vi "TestFastLocalizeCPU.vi"() -> ()   [LabVIEW 2011]
uses:
  CpuTrackDLL.vi
panel:
  out "debug":T1(plugin-control)
  out "median":sgl
  out "xcorpos":cluster{"XCor X":sgl, "XCor Y":sgl}
  out "COM":cluster{"comX":sgl, "comY":sgl}
  out "Image":T1(plugin-control)
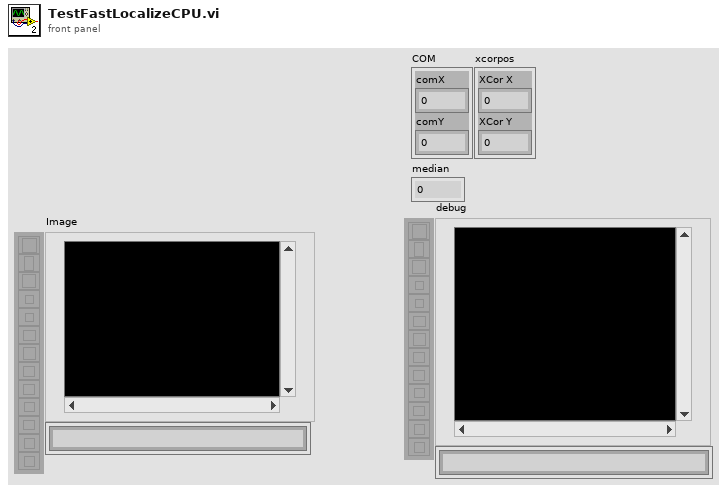
[diagram p1: front panel]
types:
  T1 = typedef "IMAQ Image.ctl" = refnum<image>
  T2 = typedef "Image Type" = u32
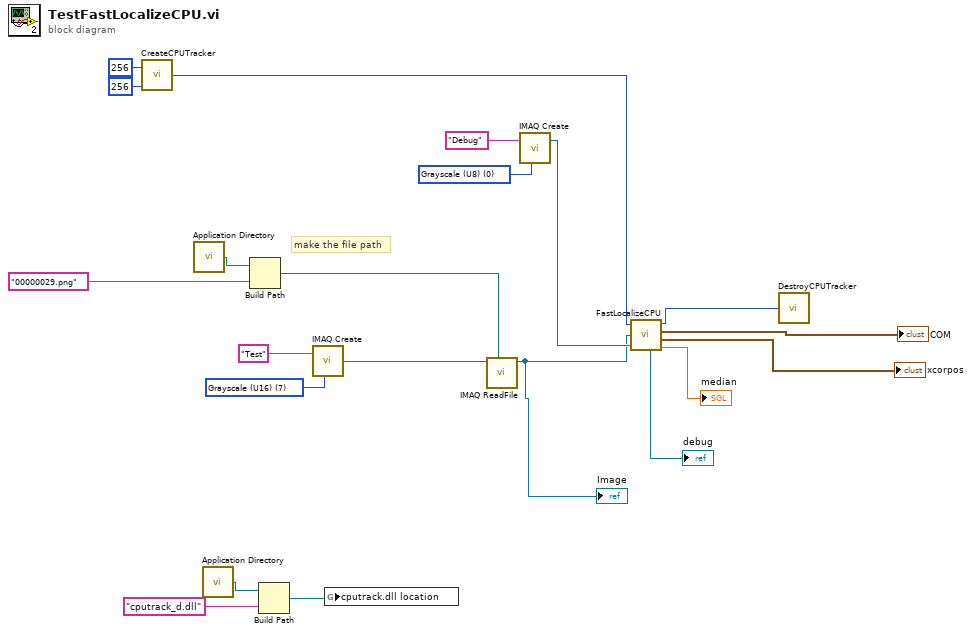
[diagram p0: block diagram]
diagram:
  w14 = T2 0 items=["Grayscale (U8)", "Grayscale (I16)", "Grayscale (SGL)", "Complex (CSG)", "RGB (U32)", "HSL (U32)", "RGB (U64)", "Grayscale (U16)"] ("Image Type")
  w16 = T2 7 items=["Grayscale (U8)", "Grayscale (I16)", "Grayscale (SGL)", "Complex (CSG)", "RGB (U32)", "HSL (U32)", "RGB (U64)", "Grayscale (U16)"] ("Image Type")
  # "make the file path"
  n1 = call "CreateCPUTracker.vi"("height"=u32 256, "width"=u32 256) -> ("return type"=w6:u64)
  n2 = call <vilib>:"Application Directory.vi"() -> ("Application Directory"=w19:path)
  n3 = call <vilib>:"Application Directory.vi"() -> ("Application Directory"=w13:path)
  n4 = Build Path(base path=w19, name or relative path="00000029.png") -> (appended path=w17:path)
  n5 = Build Path(base path=w13, name or relative path="cputrack_d.dll") -> (appended path=w11:path)
  n6 = call "IMAQ Create"("Image Name"="Test" ("String"), "Image Type"=w16) -> ("New Image"=w20:T1)  [unwired: 3 in, 1 out]
  n7 = global write "CpuTrackDLL.vi" "cputrack.dll location"(w11) -> ()
  n8 = call "IMAQ ReadFile"("File Path"=w17, "Image"=w20) -> ("Image Out"=w7:T1)  [unwired: 5 in, 4 out]
  "Image" <- w7
  n9 = call "IMAQ Create"("Image Name"="Debug" ("String"), "Image Type"=w14) -> ("New Image"=w8:T1)  [unwired: 3 in, 1 out]
  n10 = call "FastLocalizeCPU.vi"("tracker"=w6, "input image"=w7, "debug image"=w8) -> ("tracker"=w5:u64, "COM"=→"COM":cluster{"comX":sgl, "comY":sgl}, "debug image"=→"debug":T1, "xcorpos"=→"xcorpos":cluster{"XCor X":sgl, "XCor Y":sgl}, "median"=→"median":sgl)  [unwired: 3 in]
  n11 = call "DestroyCPUTracker.vi"("tracker"=w5) -> ()
